vi "buzzer.vi"() -> ()   [LabVIEW 2013]
uses:
  <vilib>/LabVIEW Interface for Arduino/Type Defs/Pin Mode.ctl
  <vilib>/LabVIEW Interface for Arduino/LabVIEW Interface for Arduino.lvlib
panel:
  in  "Boolean":bool
  in  "Digital I/O Pin":u8
  in  "stop":bool
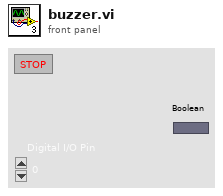
[diagram p1: front panel]
types:
  T1 = typedef "LabVIEW Interface for Arduino.lvlib/Pin Mode.ctl" = enum8{"Input", "Output"}
  T2 = typedef "LabVIEW Interface for Arduino.lvlib/Arduino Resource.ctl" = cluster{"VISA resource":refnum<visa-resource-name>, "Board Type":T3, "Connection Type":enum8{"USB / Serial"}, "Bytes Per Packet (15)":u8}
  T3 = typedef "LabVIEW Interface for Arduino.lvlib/Board Type.ctl" = enum16{"Uno", "Dimuelanove w/Atmega 328", "Mega 2560"}
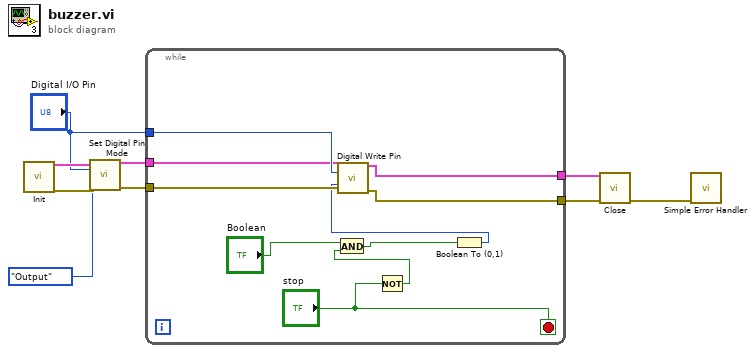
[diagram p0: block diagram]
diagram:
  n1 = call <vilib>:"Init.vi"() -> ("Arduino Resource"=w9:T2, "error out"=w8:errorcluster)  [unwired: 18 in]
  n2 = call <vilib>:"Set Digital Pin Mode.vi"("Arduino Resource"=w9, "Digital I/O Pin"="Digital I/O Pin", "Pin Mode (Input)"=Pin_Mode."Output", "error in"=w8) -> ("Arduino Resource"=w2:T2, "error out"=w4:errorcluster)  [unwired: 10 in]
  n3 = while {
    tunnel: "Digital I/O Pin" -> [w19]
    tunnel: w4 -> [w18]
    tunnel: [w17] -> w3
    tunnel: w2 -> [w16]
    tunnel: [w15] -> w1
    stop <- "stop" stop-if-true
    n4 = Not(x="stop") -> (.not. x?=w12:bool)
    n5 = And(x="Boolean", y=w12) -> (x .and. y?=w11:bool)
    n6 = Boolean To (0,1)(Boolean=w11) -> (0, 1=w10:i16)
    n7 = call <vilib>:"Digital Write Pin.vi"("Arduino Resource"=w16, "Digital I/O Pin (0)"=w19, "Value (0)"=w10, "error in"=w18) -> ("Arduino Resource"=w15:T2, "error out"=w17:errorcluster)  [unwired: 10 in]
  }
  n8 = call <vilib>:"Close.vi"("Arduino Resource"=w1, "error in"=w3) -> ("error out"=w7:errorcluster)  [unwired: 13 in]
  n9 = call <vilib>:"Simple Error Handler.vi"("error in (no error)"=w7) -> ()  [unwired: 4 in, 5 out]
